vi "test_CCDRestartTEST.vi"(6 "Delay between send and receive [ms]":i32=100, 7 "Test should pass":bool=TRUE, 8 "error in":errorcluster, 9 "tear down connection":bool=TRUE, 10 "set-up a connection":bool=TRUE, 11 "device selection":enum16{"monochromator", "CCD", "SCD"}(ring)=enum."CCD") -> (0 "error out":errorcluster)   [LabVIEW 2023]
uses:
  Classes/CCD/CCD.lvclass
  <vilib>/addons/_JKI Toolkits/Caraya/classes/Assert/Assert Not Error.vi
  <vilib>/addons/_JKI Toolkits/Caraya/classes/Test/Test.lvclass
  <vilib>/addons/_JKI Toolkits/Caraya/classes/Assert/Assert.lvclass
  <vilib>/addons/_JKI Toolkits/Caraya/classes/Assert/Assert Error.vi
  C:/Users/grju/Desktop/AbgelegteDokumente/Kunden/Horiba/horiba-labview-sdk/Source/Classes/GenericDevice/GenericDevice.lvclass
  C:/Users/grju/Desktop/AbgelegteDokumente/Kunden/Horiba/horiba-labview-sdk/Source/Classes/CCD/CCD.lvclass
panel:
  # "Connector Pane"
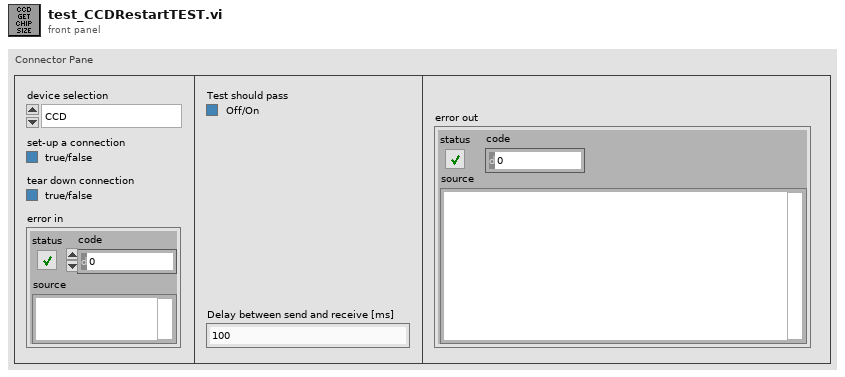
[diagram p1: front panel]
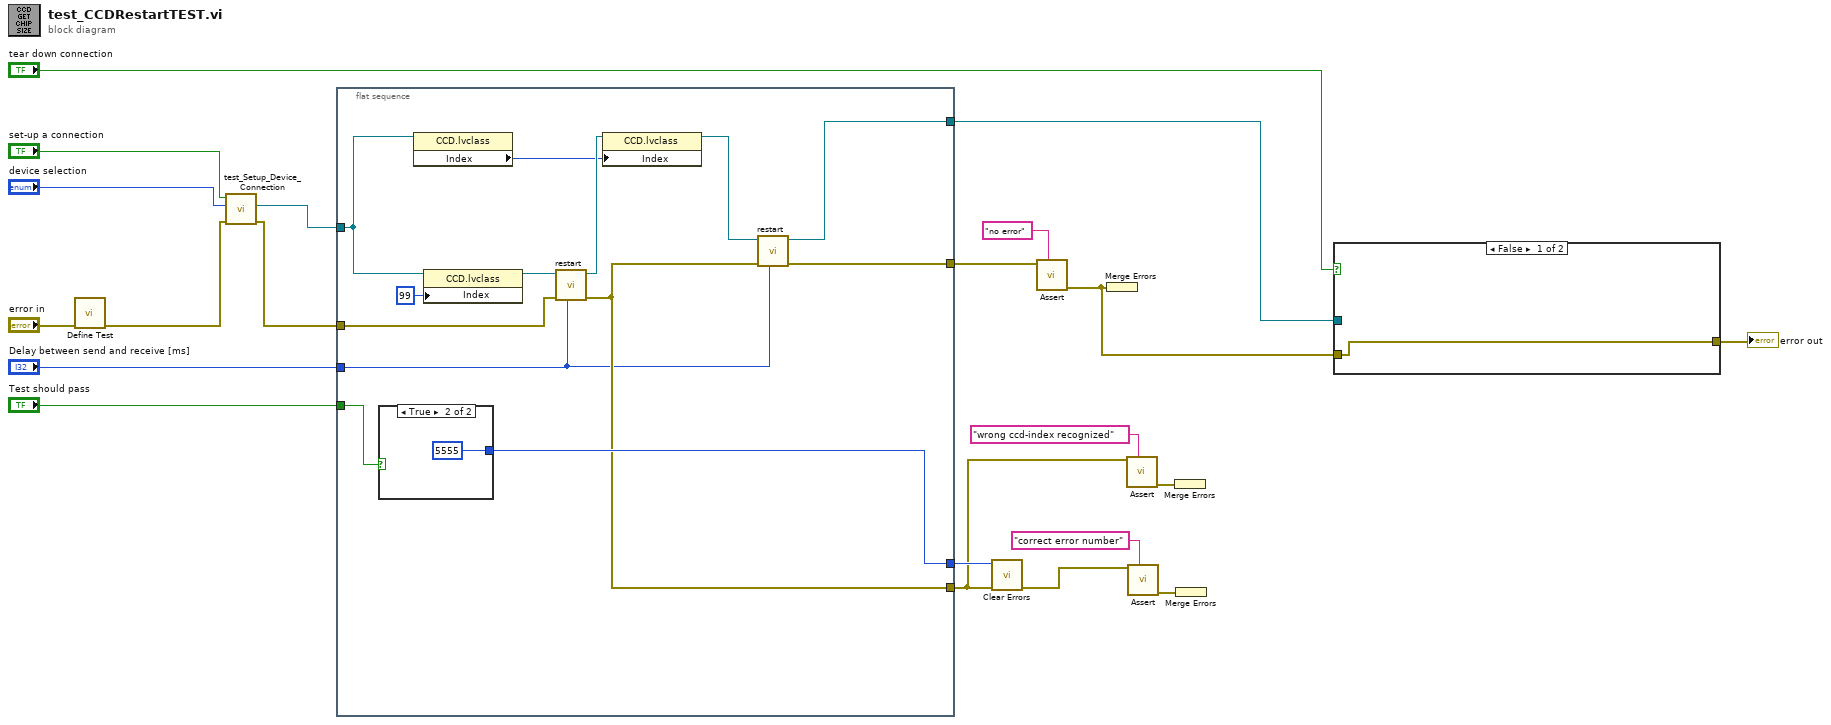
[diagram p0: block diagram]
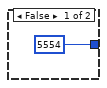
[diagram p2: hidden frame]
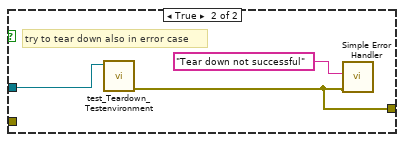
[diagram p3: hidden frame]
diagram:
  n1 = call <vilib>:"Define Test.vi"("error in (no error)"="error in") -> ("error out"=w11:errorcluster)  [unwired: 9 in, 1 out]
  n2 = call "test_Setup_Device_Connection.vi"("error in (no error)"=w11, "device selection"="device selection", "set-up a connection"="set-up a connection") -> ("error out"=w9:errorcluster, "CCD.lvclass"=w10:refnum<class "CCD.lvclass">)  [unwired: 5 in, 2 out]
  n3 = flat-sequence {
    tunnel: w9 -> [w34]
    tunnel: w10 -> [w32]
    tunnel: [w24] -> w3
    tunnel: "Test should pass" -> [w33]
    tunnel: [w26] -> w15
    tunnel: "Delay between send and receive [ms]" -> [w23]
    tunnel: [w25] -> w7
    tunnel: [w22] -> w2
    frame #0 {
      n4 = case shown="True" w33 {
        tunnel: [5554 5555] -> w25
        frame False {
        }
        frame True {
        }
      }
      n5 = property class="CCD.lvclass"(reference=w32) -> ("Index"=w28:i32)  [unwired: 1 in, 2 out]
      n6 = property class="CCD.lvclass"(reference=w32, "Index"=99) -> (reference out=w31:refnum<class "CCD.lvclass">)  [unwired: 1 in, 1 out]
      n7 = call "restart.vi"("Delay between send and receive [ms]"=w23, "error in (no error)"=w34, "CCD in"=w31) -> ("error out"=w24:errorcluster, "CCD out"=w29:refnum<class "CCD.lvclass">)  [unwired: 5 in, 2 out]
      n8 = property class="CCD.lvclass"(reference=w29, "Index"=w28) -> (reference out=w27:refnum<class "CCD.lvclass">)  [unwired: 1 in, 1 out]
      n9 = call "restart.vi"("Delay between send and receive [ms]"=w23, "error in (no error)"=w24, "CCD in"=w27) -> ("error out"=w22:errorcluster, "CCD out"=w26:refnum<class "CCD.lvclass">)  [unwired: 5 in, 2 out]
    }
  }
  n10 = call <vilib>:"Clear Errors.vi"("error in (no error)"=w3, "specific error code to clear (0: all)"=w7) -> ("error out"=w6:errorcluster)  [unwired: 4 in, 1 out]
  n11 = call-poly <vilib>:"Assert.vi"("Label"="no error" ("Label (VI Title)"), "Not Error?"=w2) -> ("error out"=w1:errorcluster)  [unwired: 8 in, 1 out]
  n12 = Merge Errors(w1) -> ()  [unwired: 1 out]
  n13 = call-poly <vilib>:"Assert.vi"("Label"="wrong ccd-index recognized" ("Label (VI Title)"), "Error?"=w3) -> ("error out"=w5:errorcluster)  [unwired: 8 in, 1 out]
  n14 = call-poly <vilib>:"Assert.vi"("Label"="correct error number" ("Label (VI Title)"), "Not Error?"=w6) -> ("error out"=w17:errorcluster)  [unwired: 8 in, 1 out]
  n15 = Merge Errors(w5) -> ()  [unwired: 1 out]
  n16 = Merge Errors(w17) -> ()  [unwired: 1 out]
  n17 = case shown="False" "tear down connection" {
    tunnel: w15 -> [_ w39]
    tunnel: [w37 w38] -> w14
    tunnel: w1 -> [w37 _]
    frame False {
    }
    frame True {
      # "try to tear down also in error case"
      n18 = call "test_Teardown_Testenvironment.vi"("GenericDevice.lvclass"=w39) -> ("error out"=w38:errorcluster)  [unwired: 9 in, 1 out]
      n19 = call <vilib>:"Simple Error Handler.vi"("error source (\" \")"="Tear down not successful" ("error source (\" \")"), "error in (no error)"=w38) -> ()  [unwired: 3 in, 5 out]
    }
  }
  "error out" <- w14
